vi "ADAM_Module_Type.vi"(1 "Module Type":T1) -> (0 "String":string)   [LabVIEW 2012]
uses:
  ADAM Controls/Module_type_ADAM.ctl
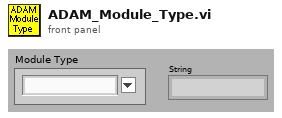
[diagram p1: front panel]
types:
  T1 = typedef "Module_type_ADAM.ctl" = string
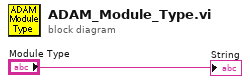
[diagram p0: block diagram]
diagram:
  "String" <- "Module Type"
